vi "Acquire Flann.vi"(8 "error in (no error)":errorcluster) -> (0 "error out":errorcluster, 3 "semaphore":T1)   [LabVIEW 2020, in "KD Tree.lvlib"]
uses:
  KD Tree.lvlib
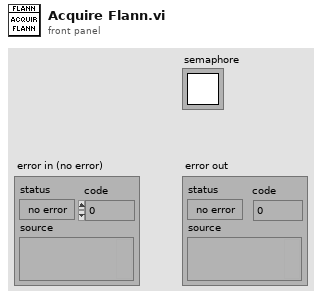
[diagram p1: front panel]
types:
  T1 = typedef "Semaphore RefNum" = refnum<k1>
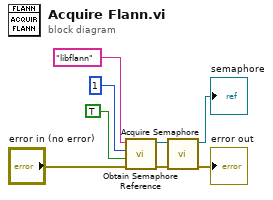
[diagram p0: block diagram]
diagram:
  n1 = call <vilib>:"Obtain Semaphore Reference.vi"("error in (no error)"="error in (no error)", "create if not found (T)"=TRUE, "size (1)"=1, "name (unnamed)"="libflann") -> ("error out"=w4:errorcluster, "semaphore"=w8:T1)  [unwired: 1 in, 1 out]
  n2 = call <vilib>:"Acquire Semaphore.vi"("error in (no error)"=w4, "semaphore"=w8) -> ("error out"=→"error out":errorcluster, "semaphore out"=→"semaphore":T1)  [unwired: 3 in, 1 out]
